vi "_ProcessDVData.vi"(3 "LastPeakHeight":dbl) -> (0 "NewPeakHeight":dbl, 1 "GotoNextStep":bool)   [LabVIEW 2012]
uses:
  Type/_Data Operation.ctl
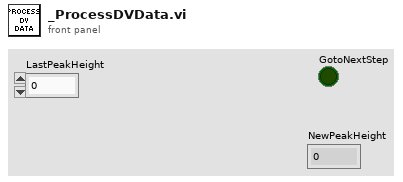
[diagram p1: front panel]
types:
  T1 = typedef "_Data Operation.ctl" = enum8{"Initialize", "Get Data", "Set Data", "Close"}
  T2 = typedef "_Current Data.ctl" = cluster{"Scan#":i32, "Run Time (mS)":i32, "TIC X":dbl[], "TIC Y":dbl[][], "MassRange":cluster{"X Title":string, "X":dbl[], "Y":i32[]}[], "Fixed Mass (amu)":dbl, "Method":T3}
  T3 = typedef "_XML Expt.ctl" = cluster{"StartT(mS)":i32, "#Cycles":i32, "PauseT(uS)":i32, "ScanType":i32, "Polarity":u8, "FixedMass":dbl, "DelayT(mS)":i32, "Active Ch":T4[], "Mass Range":T5[]}
  T4 = typedef "_XML Lens.ctl" = cluster{"Value":dbl, "ChID":u8}
  T5 = typedef "_Mass Range Property.ctl" = cluster{"Start":dbl, "Stop":dbl, "Step Size":dbl, "Steps":i32, "Dwell":dbl, "Parameters":T6[], "Res":T7}
  T6 = typedef "_Mass Range Parameters.ctl" = cluster{"Name":string, "Ch#":u8, "StartV":dbl, "StopV":dbl, "StepV":dbl, "Index":u8}
  T7 = typedef "_RT Res Type.ctl" = u16
  T8 = typedef "_Peak Property.ctl" = cluster{"Centroid":dbl, "Height":dbl, "FWHM":dbl, "Resolution":dbl, "Area":dbl, "StoN":dbl, "ApexX":dbl, "Baseline":dbl, "LEdgeX":dbl, "LEdgeY":dbl, "REdgeX":dbl, "REdgeY":dbl, "LEdgeFWHM":dbl, "REdgeFWHM":dbl}
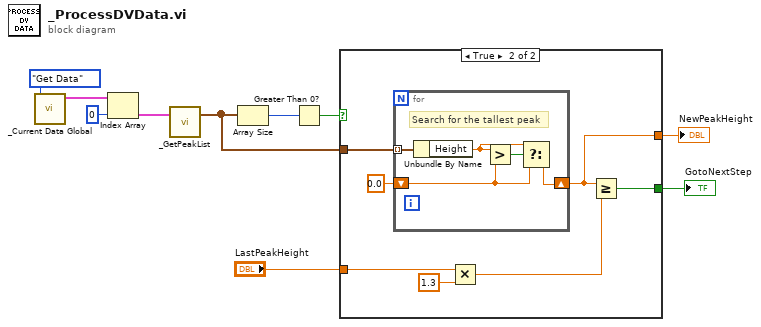
[diagram p0: block diagram]
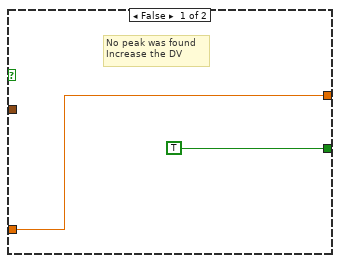
[diagram p2: hidden frame]
diagram:
  n1 = call "_Current Data Global.vi"("Operation"=_Data_Operation."Get Data") -> ("CurrentData"=w9:T2[])  [unwired: 3 in, 3 out]
  n2 = Index Array(array=w9, index=0) -> (element=w7:T2)
  n3 = call "_GetPeakList.vi"("Current Data"=w7) -> ("PeakList"=w4:T8[])  [unwired: 2 in]
  n4 = Array Size(array=w4) -> (size(s)=w6:i32)
  n5 = Greater Than 0?(x=w6) -> (x > 0?=w5:bool)
  n6 = case shown="True" w5 {
    tunnel: w4 -> [_ w18]
    tunnel: [TRUE w17] -> w3
    tunnel: "LastPeakHeight" -> [w12 w14]
    tunnel: [w12 w13] -> w1
    frame False {
      # "No peak was found\nIncrease the DV"
    }
    frame True {
      n7 = for {
        tunnel: w18 -> [w24] mode=indexing
        shift-right: [w20] -> w13
        shift-left: 0.0 -> [w21]
        # "Search for the tallest peak"
        n8 = Unbundle By Name(w24) -> ("Height"=w22:dbl)
        n9 = Greater?(x=w22, y=w21) -> (0:w23:bool)
        n10 = Select(t=w22, s=w23, f=w21) -> (s? t:f=w20:dbl)
      }
      n11 = Multiply(x=w14, y=1.3) -> (x*y=w15:dbl)
      n12 = Greater Or Equal?(x=w13, y=w15) -> (x >= y?=w17:bool)
    }
  }
  "GotoNextStep" <- w3
  "NewPeakHeight" <- w1
